vi "ExSubSpecWithCameraOpen.vi"(3 "error in (no error)":errorcluster, 4 "Grating speed":dbl format="%.2f", 5 "Grating number":i16, 6 "Camera Handle":u32) -> (0 "error out":errorcluster, 1 "Camera Handle":u32, 2 "Spectrometer Handle":u32)   [LabVIEW 2010]
panel:
  # "ExSubSpecWithCameraOpen:\nThis Sub-VI opens a spectrometer using a previously\nopened camera port, sets the grating\nand sets the speed for wavelength movement. It \nretruns a spectrometer handle. If the spectrometer\nis associated with a camera it will open it using the\ncamera handle."
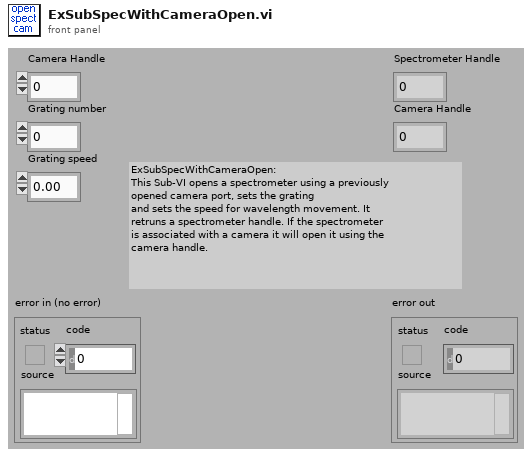
[diagram p1: front panel]
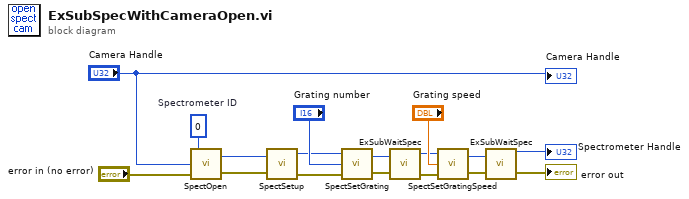
[diagram p0: block diagram]
diagram:
  w1 = u32 0  # Spectrometer ID
  n1 = call <userlib>:"SpectOpen.vi"("error in"="error in (no error)", "Camera Handle"="Camera Handle", "Spectrometer ID"=w1) -> ("error out"=w3:errorcluster, "Spectrometer Handle"=w5:u32)
  n2 = call <userlib>:"SpectSetup.vi"("error in"=w3, "Spectrometer Handle"=w5) -> ("error out"=w2:errorcluster, "Spectrometer Handle"=w4:u32)
  n3 = call <userlib>:"SpectSetGrating.vi"("error in"=w2, "Grating Number"="Grating number", "Sepctrometer Handle"=w4) -> ("error out"=w13:errorcluster, "Spectrometer Handle"=w12:u32)
  n4 = call "ExSubWaitSpec.vi"("error in (no error)"=w13, "Spectrometer Handle"=w12) -> ("error out"=w11:errorcluster, "Spectrometer handle"=w10:u32)
  n5 = call <userlib>:"SpectSetGratingSpeed.vi"("error in"=w11, "Grating Speed"="Grating speed", "Spectrometer Handle"=w10) -> ("error out"=w8:errorcluster, "Spectrometer Handle"=w9:u32)
  n6 = call "ExSubWaitSpec.vi"("error in (no error)"=w8, "Spectrometer Handle"=w9) -> ("error out"=→"error out":errorcluster, "Spectrometer handle"=→"Spectrometer Handle":u32)
  "Camera Handle" <- "Camera Handle"
